vi "test Error Propagation in Mock Transceiver.vi"(8 "error in (no error)":errorcluster, 11 "TestCase in":refnum<class "Transceiver Test Cases.lvclass">) -> (0 "error out":errorcluster, 3 "TestCase out":refnum<class "Transceiver Test Cases.lvclass">)   [LabVIEW 2017, in "Transceiver Test Cases.lvclass"]
uses:
  Transceiver Test Cases.lvclass
  Configuration/Public/Controls/DSF Engine Transfer Group Configuration.ctl
  Configuration/Public/Controls/DSF Direction.ctl
  Configuration/Public/Controls/DSF Timing Info.ctl
  Configuration/Public/Controls/DSF Engine Transfer Configuration.ctl
  Configuration/Public/Controls/DSF Byte Order.ctl
  Configuration/Public/Controls/DSF Engine Channel Configuration.ctl
  Configuration/Public/Controls/DSF Data Type.ctl
  Configuration/Public/Controls/DSF Settings Info.ctl
  MockTransceiver.lvclass
  Engine/Classes/Transfer Group/Transfer Group.lvclass
  DSF Core.lvlib
  <vilib>/addons/_JKI Toolkits/VI Tester/TestCase.llb/TestCase.lvclass
  C:/Program Files (x86)/National Instruments/LabVIEW 2017/vi.lib/addons/_JKI Toolkits/VI Tester/TestCase.llb/TestCase.lvclass
panel:
  out "propagated error out":errorcluster
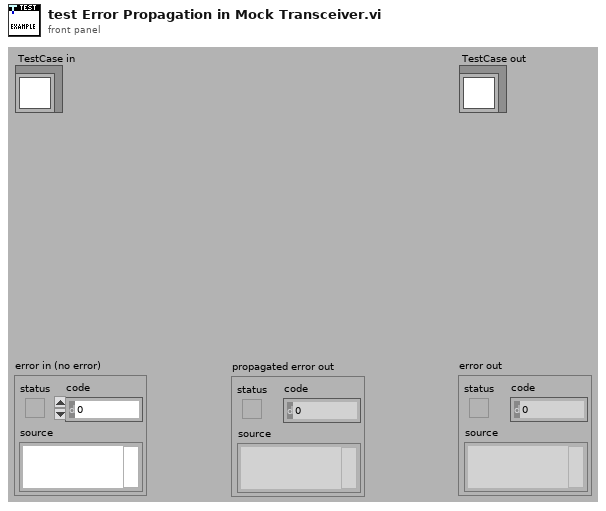
[diagram p1: front panel]
types:
  T1 = typedef "DSF Core.lvlib/DSF Settings Info.ctl" = cluster{"key":string, "value":string}[]
  T2 = typedef "DSF Core.lvlib/DSF Engine Transfer Group Configuration.ctl" = cluster{"name":string, "direction":T3, "cycle timing":T4, "Transfers":T5[], "settings":T1}
  T3 = typedef "DSF Core.lvlib/DSF Direction.ctl" = enum8{"Tx", "Rx"}
  T4 = typedef "DSF Core.lvlib/DSF Timing Info.ctl" = cluster{"priority":u64, "decimation":u64, "offset":u64}
  T5 = typedef "DSF Core.lvlib/DSF Engine Transfer Configuration.ctl" = cluster{"name":string, "byte order":T6, "channel configurations":T7[], "settings":T1}
  T6 = typedef "DSF Core.lvlib/DSF Byte Order.ctl" = enum8{"big-endian", "little-endian"}
  T7 = typedef "DSF Core.lvlib/DSF Engine Channel Configuration.ctl" = cluster{"engine offset":u64, "name":string, "data type":T8, "count":u64, "buffer offset":u64}
  T8 = typedef "DSF Core.lvlib/DSF Data Type.ctl" = enum8{"Bool", "SGL", "DBL", "I8", "I16", "I32", "I64", "U8", "U16", "U32", "U64"}
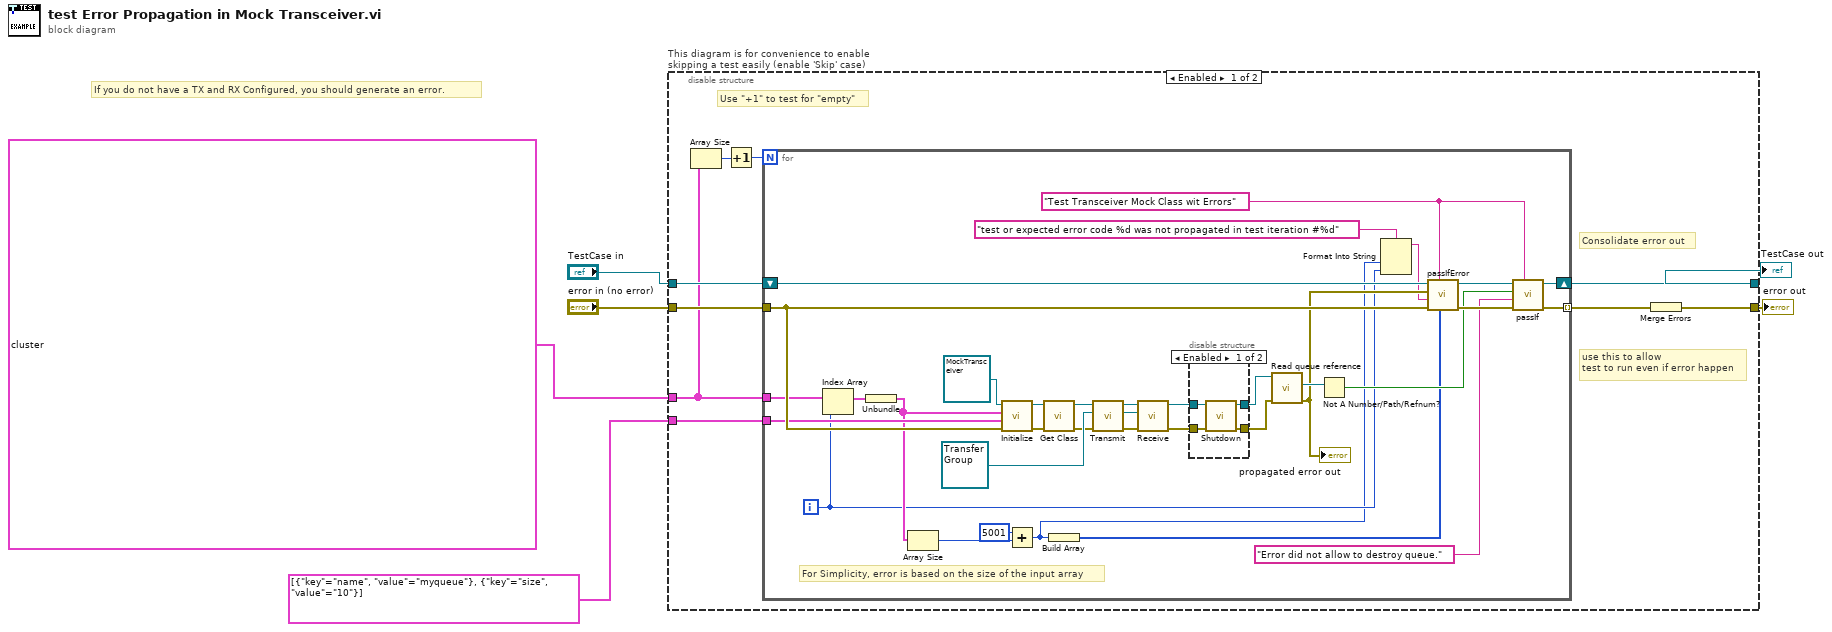
[diagram p0: block diagram]
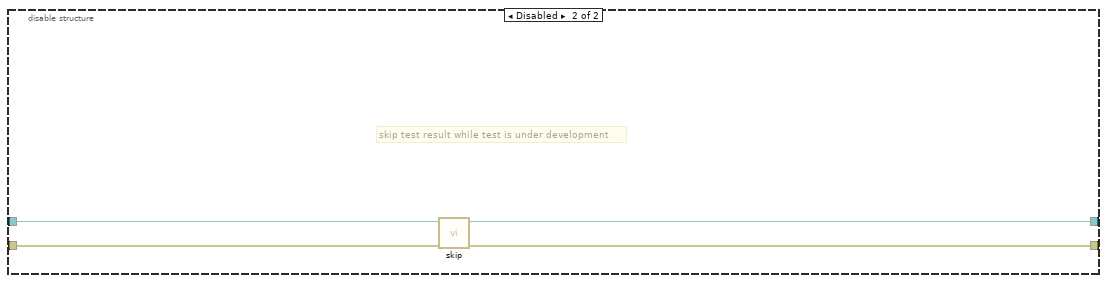
[diagram p3: hidden frame]
diagram:
  # "If you do not have a TX and RX Configured, you should generate an error."
  n1 = disable-structure "This diagram is for convenience to enable skipping a test easily (enable 'Skip' case)" shown="Enabled" {
    disable-tunnel: "TestCase in" -> [w15 w60]
    disable-tunnel: [w14 w58] -> w5
    disable-tunnel: [w7 w59] -> w4
    disable-tunnel: "error in (no error)" -> [w13 w57]
    disable-tunnel: cluster{"Transfer Groups Configurations":T2[]}[] [{"Transfer Groups Configurations"=[{"name"="", "direction"=enum."Tx", "cycle timing"={"priority"=0, "decimation"=1, "offset"=0}, "Transfers"=[], "settings"=[]}]}, {"Transfer Groups Configurations"=[{"name"="", "direction"=enum."Rx", "cycle timing"={"priority"=0, "decimation"=1, "offset"=0}, "Transfers"=[], "settings"=[]}]}, {"Transfer Groups Configurations"=[{"name"="", "direction"=enum."Tx", "cycle timing"={"priority"=0, "decimation"=1, "offset"=0}, "Transfers"=[], "settings"=[]}, {"name"="", "direction"=enum."Tx", "cycle timing"={"priority"=0, "decimation"=1, "offset"=0}, "Transfers"=[], "settings"=[]}]}, {"Transfer Groups Configurations"=[{"name"=" ", "direction"=enum."Rx", "cycle timing"={"priority"=0, "decimation"=1, "offset"=0}, "Transfers"=[], "settings"=[]}, {"name"="", "direction"=enum."Rx", "cycle timing"={"priority"=0, "decimation"=1, "offset"=0}, "Transfers"=[], "settings"=[]}]}] -> [w12 _]
    disable-tunnel: T1 [{"key"="name", "value"="myqueue"}, {"key"="size", "value"="10"}] ("transceiver settings") -> [w10 _]
    frame Enabled {
      # "Consolidate error out"
      # "use this to allow\ntest to run even if error happen"
      # "Use \"+1\" to test for \"empty\""
      n2 = Array Size(array=w12) -> (size(s)=w11:i32)
      n3 = Increment(x=w11) -> (x+1=w9:i32)
      n4 = for {
        N: w9 -> [_]
        shift-right: [w30] -> w14
        shift-left: w15 -> [w50]
        tunnel: w12 -> [w48]
        tunnel: w10 -> [w34]
        tunnel: w13 -> [w49]
        tunnel: [w32] -> w8 mode=indexing
        i -> [w17]
        w29 = "Test Transceiver Mock Class wit Errors" ("custom report message (\"\")")
        # "For Simplicity, error is based on the size of the input array"
        n5 = Index Array(array=w48, index=w17) -> (element=w47:cluster{"Transfer Groups Configurations":T2[]})
        n6 = Unbundle(w47) -> ("Transfer Groups Configurations"=w23:T2[])
        n7 = Array Size(array=w23) -> (size(s)=w22:i32)
        n8 = call-dynamic "Initialize.vi"("error in (no error)"=w49, "transceiver settings"=w34, "Transfer Groups Configurations"=w23, "MockTransceiver in"=refnum<class "MockTransceiver.lvclass"> refnum) -> ("error out"=w36:errorcluster, "MockTransceiver out"=w37:refnum<class "MockTransceiver.lvclass">)  [unwired: 6 in]
        n9 = Add(x=5001 ("code"), y=w22) -> (x+y=w16:i32)
        n10 = call-dynamic "Get Class.vi"("error in (no error)"=w36, "MockTransceiver in"=w37) -> ("error out"=w38:errorcluster, "MockTransceiver out"=w39:refnum<class "MockTransceiver.lvclass">)  [unwired: 7 in, 1 out]
        n11 = Build Array(w16) -> (w21:i32[])
        n12 = call-dynamic "Transmit.vi"("error in (no error)"=w38, "Transfer Group in"=refnum<class "Transfer Group.lvclass"> refnum, "MockTransceiver in"=w39) -> ("error out"=w40:errorcluster, "Transfer Group out"=w41:refnum<class "Transfer Group.lvclass">, "MockTransceiver out"=w42:refnum<class "MockTransceiver.lvclass">)  [unwired: 6 in]
        n13 = call-dynamic "Receive.vi"("error in (no error)"=w40, "Transfer Group in"=w41, "MockTransceiver in"=w42) -> ("error out"=w43:errorcluster, "MockTransceiver out"=w27:refnum<class "MockTransceiver.lvclass">)  [unwired: 6 in, 1 out]
        n14 = disable-structure shown="Enabled" {
          disable-tunnel: [w54 w56] -> w26
          disable-tunnel: w27 -> [w53 w56]
          disable-tunnel: w43 -> [w52 w55]
          disable-tunnel: [w51 w55] -> w35
          frame Enabled {
            n15 = call-dynamic "Shutdown.vi"("error in (no error)"=w52, "MockTransceiver in"=w53) -> ("error out"=w51:errorcluster, "MockTransceiver out"=w54:refnum<class "MockTransceiver.lvclass">)  [unwired: 8 in]
          }
          frame Disabled {
          }
        }
        n16 = call-dynamic "Read queue reference.vi"("error in (no error)"=w35, "MockTransceiver in"=w26) -> ("error out"=w25:errorcluster, "queue reference"=w46:refnum<queue>)  [unwired: 7 in, 1 out]
        "propagated error out" <- w25
        n17 = Not A Number/Path/Refnum?(number/path/refnum=w46) -> (NaN/Path/Refnum?=w24:bool)
        n18 = Format Into String(format string="test or expected error code %d was not propagated in test iteration #%d" ("custom report message (\"\")"), w16, w17) -> (resulting string=w18:string)  [unwired: 2 in, 1 out]
        n19 = call-dynamic "passIfError.vi"("passing error codes (default = any error code)"=w21, "custom report message (\"\")"=w29, "error in (no error)"=w49, "task (\"\")"=w18, "error"=w25, "TestCase in"=w50) -> ("error out"=w33:errorcluster, "TestCase out"=w31:refnum<class "Transceiver Test Cases.lvclass">)  [unwired: 4 in]
        n20 = call-dynamic "passIf.vi"("custom report message (\"\")"=w29, "error in (no error)"=w33, "message (\"\")"="Error did not allow to destroy queue." ("message (\"\")"), "pass"=w24, "TestCase in"=w31) -> ("error out"=w32:errorcluster, "TestCase out"=w30:refnum<class "Transceiver Test Cases.lvclass">)  [unwired: 5 in]
      }
      n21 = Merge Errors(w8) -> (w7:errorcluster)
    }
    frame Disabled {
      # "skip test result while test is under development"
      n22 = call <vilib>:"skip.vi"("error in (no error)"=w57, "TestCase in"=w60) -> ("error out"=w59:errorcluster, "TestCase out"=w58:refnum<class "Transceiver Test Cases.lvclass">)  [unwired: 8 in]
    }
  }
  "error out" <- w4
  "TestCase out" <- w5
